vi "mod_Phase Noise Calculation.vi"(0 "IQ data (complex)":cluster{"t0":dbl, "dt":dbl, "Y":cdb[]} {"Y" format="%.2f"; "dt" format="%.2f"; "t0" format="%.2f"}, 1 "offset stop (Hz)":dbl=1000000.0 format="%.2p", 5 "window":T2(ring)=enum."Hanning", 7 "restart averaging (F)":bool, 9 "averaging parameters":T1={"averaging mode"=enum."RMS averaging", "weighting mode"=enum."Exponential", "number of averages"=10} {"number of averages" min=1}, 11 "error in (no error)":errorcluster, 12 "desired offset values (Hz)":dbl[](array[numeric])=[1000.0, 10000.0, 100000.0] format="%.2f") -> (4 "appended array":cluster{"f0":dbl, "df":dbl, "magnitude":dbl[]}[](array[cluster]), 6 "averaging done":bool, 8 "averages completed":dbl, 10 "phase noise at actual offsets":dbl[](array[numeric]) format="%.4f", 14 "actual offset values (Hz)":dbl[](array[numeric]) format="%.2f", 15 "error out":errorcluster)   [LabVIEW 2020, in "niAMT.lvlib"]
doc: "This VI converts the IQ data (complex) in the cartesean form to the phase noise density.\n\nThis VI first converts the IQ data (complex) to the polar form. It then unwraps the phase and then performs a linear fit on the phase data. It then computes the error between the actual phase and the linear fit. It then computes a power spectral density measurement on the phase error, thus resulting in the phase noise density."
uses:
  <vilib>/addons/Modulation/niAMT.lvlib
  <vilib>/Analysis/1siggen.llb/Ramp Pattern by Samples.vi
  <vilib>/measure/maspectr.llb/FFT Power Spectral Density for 1 Chan.vi
  <vilib>/Waveform/WDTOps.llb/WDT Get XY Value DBL.vi
  <vilib>/Analysis/NI_AALPro.lvlib
  <vilib>/measure/NI_MAPro.lvlib
  <vilib>/Analysis/NI_AALBase.lvlib
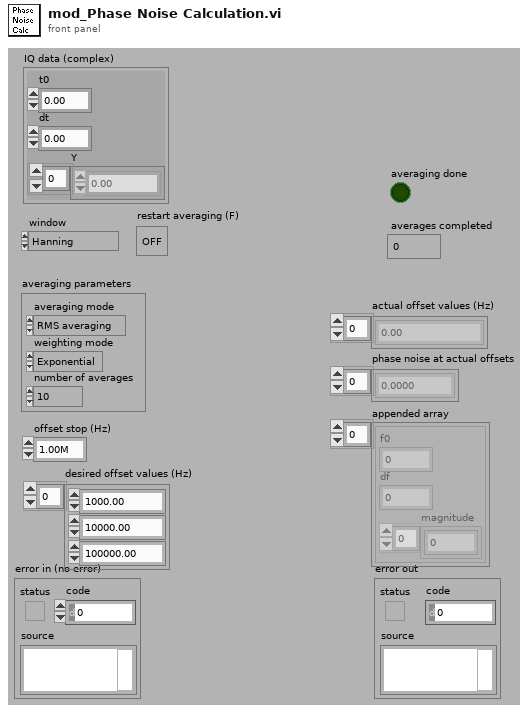
[diagram p1: front panel]
types:
  T1 = cluster{"averaging mode":enum16{"No averaging", "Vector averaging", "RMS averaging", "Peak hold"}, "weighting mode":enum16{"Linear", "Exponential"}, "number of averages":u32}
  T2 = enum16{"None ", "Hanning", "Hamming", "Blackman-Harris", "Exact Blackman", "Blackman", "Flat Top", "4 Term B-Harris ", "7 Term B-Harris", "Low Sidelobe"}
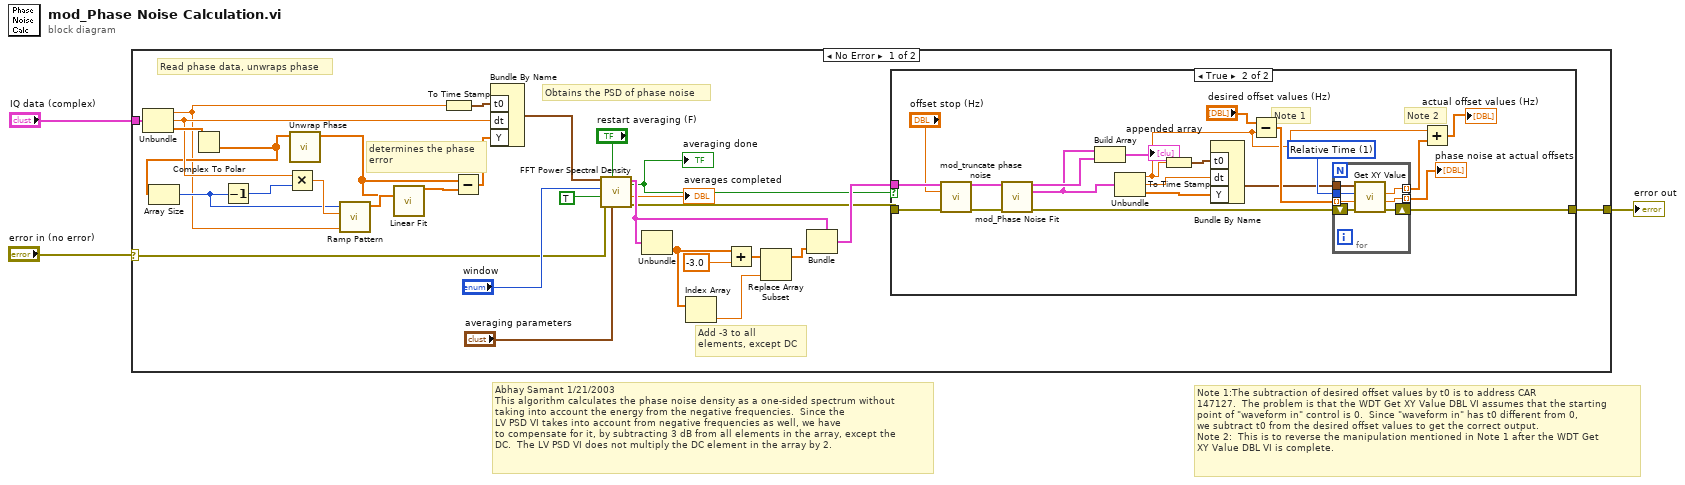
[diagram p0: block diagram]
diagram:
  # "Note 1:The subtraction of desired offset values by t0 is to address CAR \n147127.  The problem is that the WDT Get XY Value DBL VI assumes that the starting \npoint of \"waveform in\" control is 0.  Since \"waveform in\" has t0 different from 0,\nwe subtract t0 from the desired offset values to get the correct output.\nNote 2:  This is to reverse the manipulation mentioned in Note 1 after the WDT Get \nXY Value DBL VI is complete."
  # "Abhay Samant 1/21/2003\nThis algorithm calculates the phase noise density as a one-sided spectrum without \ntaking into account the energy from the negative frequencies.  Since the\nLV PSD VI takes into account from negative frequencies as well, we have \nto compensate for it, by subtracting 3 dB from all elements in the array, except the\nDC.  The LV PSD VI does not multiply the DC element in the array by 2."
  n1 = case shown="No Error" "error in (no error)" {
    selector: "error in (no error)" -> [w4 w63]
    tunnel: "IQ data (complex)" -> [w27 _]
    tunnel: [w8 w63] -> w1
    frame No Error {
      # "Add -3 to all\nelements, except DC"
      # "Obtains the PSD of phase noise"
      # "determines the phase \nerror"
      # "Read phase data, unwraps phase"
      n2 = Unbundle(w27) -> ("t0"=w10:dbl, "dt"=w24:dbl, "Y"=w26:cdb[])
      n3 = Complex To Polar(r * e^(i*theta)=w26) -> (theta=w23:dbl[])  [unwired: 1 out]
      n4 = Array Size(array=w23) -> (size(s)=w28:i32)
      n5 = Decrement(x=w28) -> (x-1=w32:i32)
      n6 = Multiply(x=w24, y=w32) -> (x*y=w31:dbl)
      n7 = call <vilib>:"Unwrap Phase.vi"("Phase"=w23) -> ("Unwrapped Phase"=w29:dbl[])  [unwired: 1 in, 9 out]
      n8 = call-poly <vilib>:"Ramp Pattern.vi"("start"=w10, "end"=w31, "samples"=w28) -> ("Ramp Pattern"=w30:dbl[])  [unwired: 7 in, 1 out]
      n9 = call <vilib>:"Linear Fit.vi"("Y"=w29, "X"=w30) -> ("Best Linear Fit"=w33:dbl[])  [unwired: 4 in, 9 out]
      n10 = To Time Stamp(1:w10) -> (0:w9:timestamp)
      n11 = Subtract(x=w29, y=w33) -> (x-y=w25:dbl[])
      n12 = Bundle By Name("t0"=w9, "dt"=w24, "Y"=w25) -> (w22:waveform(dbl))  [unwired: 1 out]
      n13 = call-poly <vilib>:"FFT Power Spectral Density.vi"("averaging parameters"="averaging parameters", "restart averaging (F)"="restart averaging (F)", "error in (no error)"=w4, "dB On (F)"=TRUE, "window"="window", "time signal"=w22) -> ("error out"=w6:errorcluster, "averages completed"=→"averages completed":dbl, "power spectral density"=w13:cluster{"f0":dbl, "df":dbl, "magnitude":dbl[]}, "averaging done"=w5:bool)  [unwired: 2 out]
      "averaging done" <- w5
      n14 = Unbundle(w13) -> ("magnitude"=w17:dbl[])  [unwired: 2 out]
      n15 = Index Array(array=w17) -> (element=w14:dbl)  [unwired: 1 in]
      n16 = Add(x=w17, y=-3.0) -> (x+y=w15:dbl[])
      n17 = Replace Array Subset(array=w15, new element=w14) -> (w12:dbl[])  [unwired: 1 in]
      n18 = Bundle(cluster=w13, "magnitude"=w12) -> (w7:cluster{"f0":dbl, "df":dbl, "magnitude":dbl[]})  [unwired: 2 out]
      n19 = case shown="True" w5 {
        tunnel: w7 -> [_ w46]
        tunnel: w6 -> [w34 w48]
        tunnel: [w34 w54] -> w8
        frame False {
        }
        frame True {
          w55 = u16 1 items=["Index", "Relative Time"] ("mode")
          # "Note 1"
          # "Note 2"
          n20 = call <vilib>:"mod_truncate phase noise.vi"("phase noise in"=w46, "offset stop (Hz)"="offset stop (Hz)", "error in (no error)"=w48) -> ("phase noise out (truncated)"=w45:cluster{"f0":dbl, "df":dbl, "magnitude":dbl[]}, "error out"=w47:errorcluster)  [unwired: 11 out]
          n21 = call <vilib>:"mod_Phase Noise Fit.vi"("single sided phase noise density"=w45, "error in (no error)"=w47) -> ("raw phase noise"=w50:cluster{"f0":dbl, "df":dbl, "magnitude":dbl[]}, "fitted phase noise"=w49:cluster{dbl, dbl, dbl[]}, "error out"=w51:errorcluster)  [unwired: 11 out]
          n22 = Build Array(w49, w50) -> (→"appended array":cluster{"f0":dbl, "df":dbl, "magnitude":dbl[]}[])
          n23 = Unbundle(w49) -> (w36:dbl, w35:dbl, w52:dbl[])
          n24 = To Time Stamp(1:w36) -> (0:w44:timestamp)
          n25 = Bundle By Name("t0"=w44, "dt"=w35, "Y"=w52) -> (w37:waveform(dbl))  [unwired: 1 out]
          n26 = Subtract(x="desired offset values (Hz)", y=w36) -> (x-y=w40:dbl[])
          n27 = for {
            tunnel: w37 -> [w62]
            tunnel: w55 -> [w61]
            shift-right: [w59] -> w54
            shift-left: w51 -> [w60]
            tunnel: w40 -> [w58] mode=indexing
            tunnel: [w57] -> w53 mode=indexing
            tunnel: [w56] -> w39 mode=indexing
            n28 = call-poly <vilib>:"Get XY Value.vi"("error in (no error)"=w60, "Y position"=w58, "Y position format"=w61, "waveform in"=w62) -> ("error out"=w59:errorcluster, "Y value"=w57:dbl, "actual Y position"=w56:dbl)  [unwired: 5 out]
          }
          "phase noise at actual offsets" <- w53
          n29 = Add(x=w36, y=w39) -> (x+y=→"actual offset values (Hz)":dbl[])
        }
      }
    }
    frame Error {
    }
  }
  "error out" <- w1
